vi "Read Diameter Abort.vi"(8 "error in (no error)":errorcluster, 11 "IA Test Parameters in":refnum<class "IA Test Parameters.lvclass">) -> (0 "error out":errorcluster, 2 "diameter abort (mm)":dbl=70.0, 3 "IA Test Parameters out":refnum<class "IA Test Parameters.lvclass">)   [LabVIEW 2020, in "IA Test Parameters.lvclass"]
uses:
  IA Test Parameters.lvclass
  IA Test Parameters.lvclass/IA Test Parameters.ctl
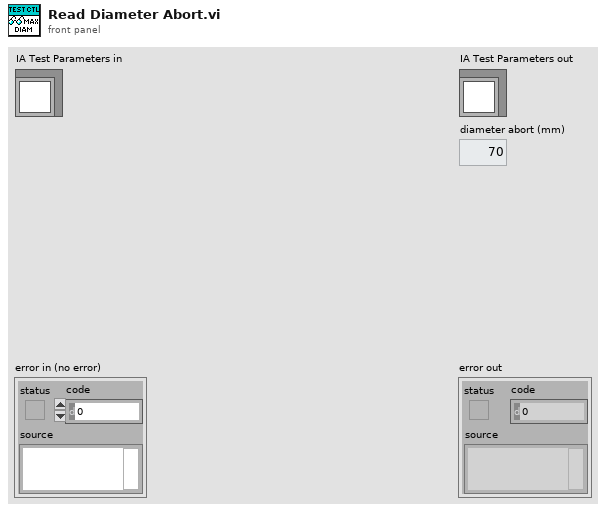
[diagram p1: front panel]
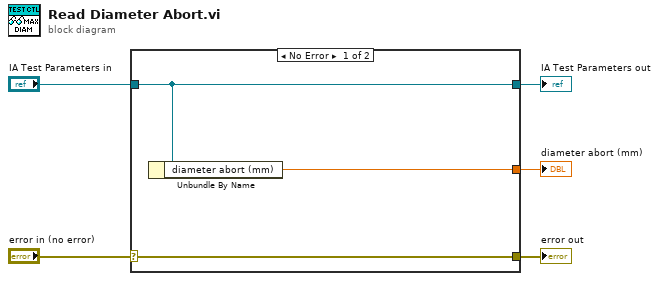
[diagram p0: block diagram]
diagram:
  n1 = case shown="No Error" "error in (no error)" {
    selector: "error in (no error)" -> [w8 w9]
    tunnel: [w8 w9] -> w4
    tunnel: [w7 w10] -> w2
    tunnel: "IA Test Parameters in" -> [w7 w10]
    tunnel: [w6 _] -> w1
    frame No Error {
      n2 = Unbundle By Name(w7) -> ("diameter abort (mm)"=w6:dbl)
    }
    frame Error {
    }
  }
  "error out" <- w4
  "IA Test Parameters out" <- w2
  "diameter abort (mm)" <- w1
